vi "FPGA SPI Command.vi"(8 "error in":errorcluster, 10 "Array":string[](array[string])) -> (0 "error out":errorcluster)   [LabVIEW 2012]
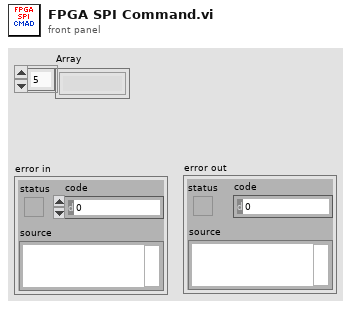
[diagram p1: front panel]
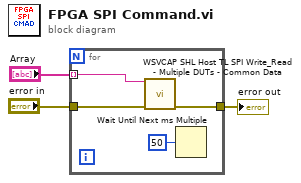
[diagram p0: block diagram]
diagram:
  n1 = for {
    tunnel: "error in" -> [w7]
    tunnel: [w6] -> w2
    tunnel: "Array" -> [w4] mode=indexing
    n2 = call "WSVCAP SHL Host TL SPI Write_Read - Multiple DUTs - Common Data.vi"("Data Out"=w4, "error in"=w7) -> ("error out"=w6:errorcluster)  [unwired: 12 in, 1 out]
    n3 = Wait Until Next ms Multiple(millisecond multiple=u32 50) -> ()  [unwired: 1 out]
  }
  "error out" <- w2
